vi "linear interp.vi"(1 "x array":dbl[](array[numeric]) format="%.4f", 2 "X data":dbl[](array[numeric]) format="%.4f", 3 "Y data":dbl[](array[numeric]) format="%.4f") -> (0 "y":dbl[](array[numeric]) format="%.4f")   [LabVIEW 2018]
panel:
  out "plotted data":cluster{dbl[], "Y data":dbl[]}[](graph)
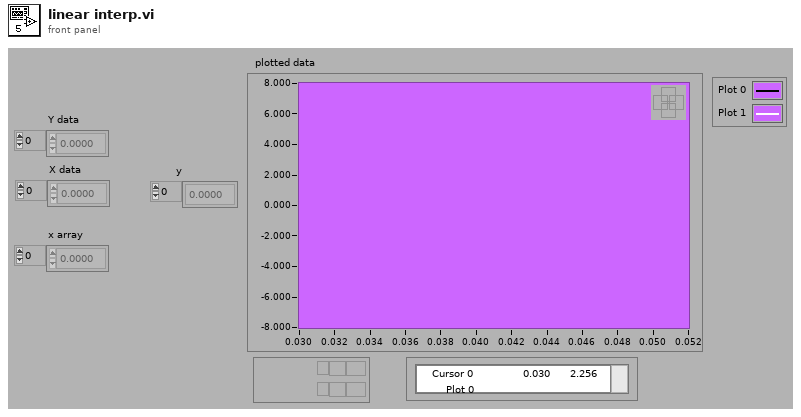
[diagram p1: front panel]
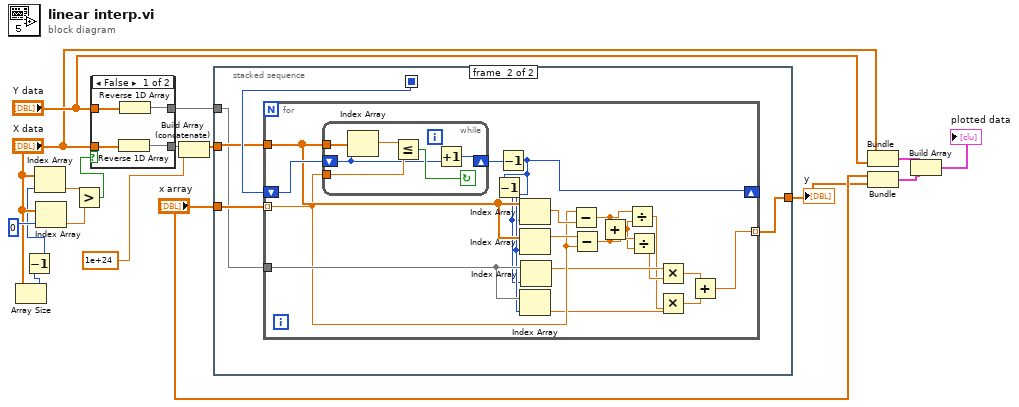
[diagram p0: block diagram]
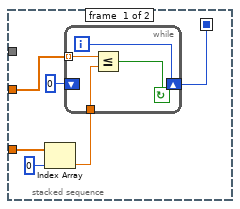
[diagram p3: hidden frame]
diagram:
  n1 = Array Size(array="X data") -> (size(s)=w2:i32)
  n2 = Decrement(x=w2) -> (x-1=w1:i32)
  n3 = Index Array(array="X data", index=w1) -> (element=w15:dbl)
  n4 = Index Array(array="X data", index=0) -> (element=w14:dbl)
  n5 = Greater?(x=w15, y=w14) -> (0:w13:bool)
  n6 = case shown="False" w13 {
    tunnel: [w20 w23] -> w12
    tunnel: "Y data" -> [w21 w23]
    tunnel: [w18 w22] -> w10
    tunnel: "X data" -> [w19 w22]
    frame False {
      n7 = Reverse 1D Array(array=w19) -> (reversed array=w18:dbl[])
      n8 = Reverse 1D Array(array=w21) -> (reversed array=w20:dbl[])
    }
    frame True {
    }
  }
  n9 = Build Array (concatenate)(w10, 1e+24) -> (w9:dbl[])
  n10 = stacked-sequence {
    seq-local: [w24 _] -> [_ w38]
    tunnel: "x array" -> [w29 w36]
    tunnel: w12 -> [_ w35]
    tunnel: w9 -> [w27 w37]
    tunnel: [_ w34] -> w11
    frame #0 {
      n11 = Index Array(array=w29, index=0) -> (element=w26:dbl)
      n12 = while {
        shift-left: 0 -> [_]
        shift-right: [w30] -> w24
        tunnel: w26 -> [w31]
        tunnel: w27 -> [w32] mode=indexing
        i -> [w30]
        stop <- w33 continue-if-true
        n13 = Less Or Equal?(x=w32, y=w31) -> (x <= y?=w33:bool)
      }
    }
    frame #1 {
      n14 = for {
        shift-right: [w53] -> _
        shift-left: w38 -> [w57]
        tunnel: w37 -> [w55]
        tunnel: w36 -> [w49] mode=indexing
        tunnel: w35 -> [w54]
        tunnel: [w41] -> w34 mode=indexing
        n15 = while {
          tunnel: w55 -> [w60]
          shift-left: w57 -> [w59]
          shift-right: [w63] -> w56
          tunnel: w49 -> [w62]
          stop <- w61 continue-if-true
          n16 = Index Array(array=w60, index=w59) -> (element=w58:dbl)
          n17 = Less Or Equal?(x=w58, y=w62) -> (x <= y?=w61:bool)
          n18 = Increment(x=w59) -> (x+1=w63:i32)
        }
        n19 = Decrement(x=w56) -> (x-1=w53:i32)
        n20 = Decrement(x=w53) -> (x-1=w52:i32)
        n21 = Index Array(array=w55, index=w52) -> (element=w51:dbl)
        n22 = Index Array(array=w55, index=w53) -> (element=w50:dbl)
        n23 = Index Array(array=w54, index=w53) -> (element=w44:dbl)
        n24 = Index Array(array=w54, index=w52) -> (element=w45:dbl)
        n25 = Subtract(x=w49, y=w51) -> (x-y=w48:dbl)
        n26 = Subtract(x=w50, y=w49) -> (x-y=w47:dbl)
        n27 = Add(x=w48, y=w47) -> (x+y=w46:dbl)
        n28 = Divide(x=w48, y=w46) -> (x/y=w39:dbl)
        n29 = Divide(x=w47, y=w46) -> (x/y=w40:dbl)
        n30 = Multiply(x=w45, y=w40) -> (x*y=w43:dbl)
        n31 = Multiply(x=w44, y=w39) -> (x*y=w42:dbl)
        n32 = Add(x=w43, y=w42) -> (x+y=w41:dbl)
      }
    }
  }
  "y" <- w11
  n33 = Bundle("X data"="X data", "Y data"="Y data") -> (w6:cluster{"X data":dbl[], "Y data":dbl[]})  [unwired: 1 in]
  n34 = Bundle("x array"="x array", w11) -> (w5:cluster{"x array":dbl[], dbl[]})  [unwired: 1 in]
  n35 = Build Array(w6, w5) -> (→"plotted data":cluster{"x array":dbl[], "Y data":dbl[]}[])
